vi "Read name.vi"(8 "error in (no error)":errorcluster, 11 "Material-Scheme in":refnum<class "Material-Scheme.lvclass">) -> (0 "error out":errorcluster, 2 "name":string, 3 "Material-Scheme out":refnum<class "Material-Scheme.lvclass">)   [LabVIEW 2024, in "TSC Material Theme.lvlib" / "Material-Scheme.lvclass"]
uses:
  Material-Scheme.lvclass
  Material-Scheme.lvclass/Material-Scheme.ctl
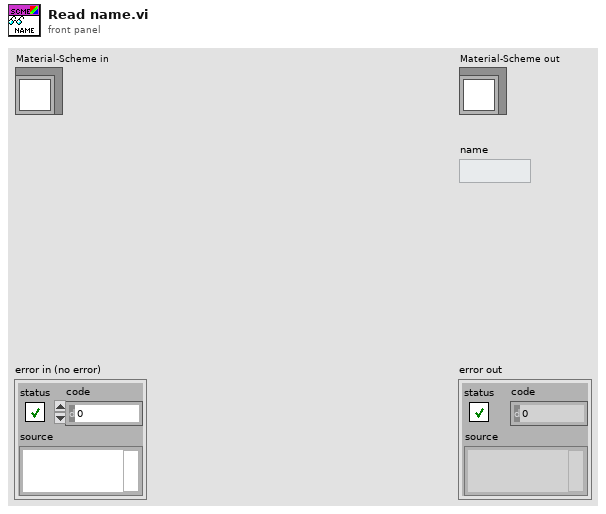
[diagram p1: front panel]
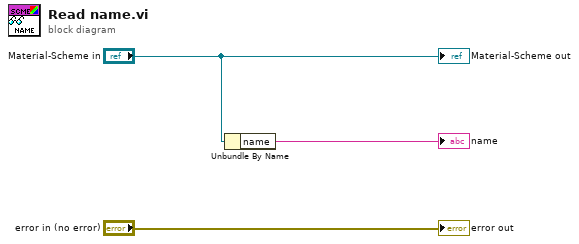
[diagram p0: block diagram]
diagram:
  n1 = Unbundle By Name("Material-Scheme in") -> ("name"=→"name":string)
  "error out" <- "error in (no error)"
  "Material-Scheme out" <- "Material-Scheme in"
